vi "CG Fehler auswahl.vi"(11 "DO 0-31":T1) -> (3 "Boolesch":bool)   [LabVIEW 2020, in "Stoermeldungen.lvlib"]
uses:
  Stoermeldungen.lvlib
  Verwaltung/Digital Ausgaenge 0-31.ctl
  Verwaltung/Verwaltung - cRIO.lvlib
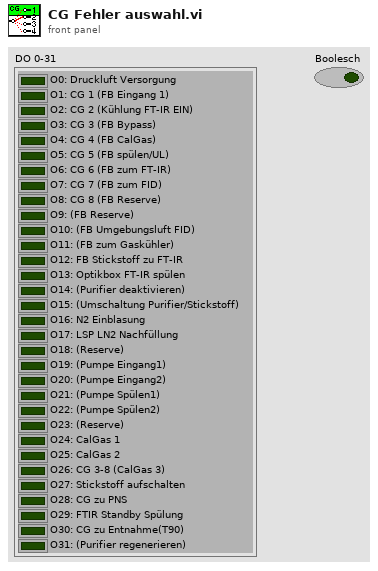
[diagram p1: front panel]
types:
  T1 = typedef "Verwaltung - cRIO.lvlib/Digital Ausgaenge 0-31.ctl" = cluster{"O0: Druckluft Versorgung":bool, "O1: CG 1 (FB Eingang 1)":bool, "O2: CG 2 (Kühlung FT-IR EIN)":bool, "O3: CG 3 (FB Bypass)":bool, "O4: CG 4 (FB CalGas)":bool, "O5: CG 5 (FB spülen/UL)":bool, "O6: CG 6 (FB zum FT-IR)":bool, "O7: CG 7 (FB zum FID)":bool, "O8: CG 8 (FB Reserve)":bool, "O9: (FB Reserve)":bool, "O10: (FB Umgebungsluft FID)":bool, "O11: (FB zum Gaskühler)":bool, "O12: FB Stickstoff zu FT-IR":bool, "O13: Optikbox FT-IR spülen":bool, "O14: (Purifier deaktivieren)":bool, "O15: (Umschaltung Purifier/Stickstoff)":bool, "O16: N2 Einblasung":bool, "O17: LSP LN2 Nachfüllung":bool, "O18: (Reserve)":bool, "O19: (Pumpe Eingang1)":bool, "O20: (Pumpe Eingang2)":bool, "O21: (Pumpe Spülen1)":bool, "O22: (Pumpe Spülen2)":bool, "O23: (Reserve)":bool, "O24: CalGas 1":bool, "O25: CalGas 2":bool, "O26: CG 3-8 (CalGas 3)":bool, "O27: Stickstoff aufschalten":bool, "O28: CG zu PNS":bool, "O29: FTIR Standby Spülung":bool, "O30: CG zu Entnahme(T90)":bool, "O31: (Purifier regenerieren)":bool}
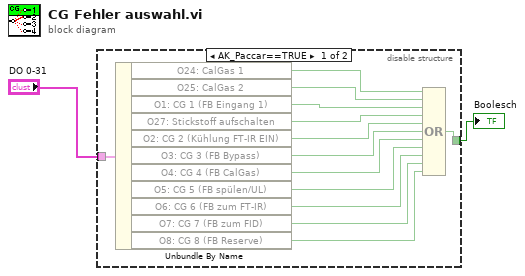
[diagram p0: block diagram]
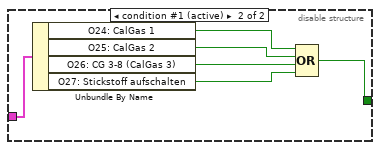
[diagram p2: hidden frame]
diagram:
  n1 = disable-structure shown="AK_Paccar==TRUE" {
    disable-tunnel: "DO 0-31" -> [w15 w21]
    disable-tunnel: [w12 w18] -> w1
    frame condition #0 {
      n2 = Unbundle By Name(w15) -> ("O24: CalGas 1"=w14:bool, "O25: CalGas 2"=w13:bool, "O1: CG 1 (FB Eingang 1)"=w10:bool, "O27: Stickstoff aufschalten"=w11:bool, "O2: CG 2 (Kühlung FT-IR EIN)"=w9:bool, "O3: CG 3 (FB Bypass)"=w8:bool, "O4: CG 4 (FB CalGas)"=w7:bool, "O5: CG 5 (FB spülen/UL)"=w6:bool, "O6: CG 6 (FB zum FT-IR)"=w5:bool, "O7: CG 7 (FB zum FID)"=w4:bool, "O8: CG 8 (FB Reserve)"=w3:bool)
      n3 = Compound Arithmetic op=OR ("Mehrfacharithmetik")(w14, w13, w10, w11, w9, w8, w7, w6, w5, w4, w3) -> (w12:bool)
    }
    frame condition #1 (active) {
      n4 = Unbundle By Name(w21) -> ("O24: CalGas 1"=w20:bool, "O25: CalGas 2"=w19:bool, "O26: CG 3-8 (CalGas 3)"=w16:bool, "O27: Stickstoff aufschalten"=w17:bool)
      n5 = Compound Arithmetic op=OR ("Mehrfacharithmetik")(w20, w19, w16, w17) -> (w18:bool)
    }
  }
  "Boolesch" <- w1
